vi "Read Element of Array.vi"(8 "error in (no error)":errorcluster, 10 "index":i32, 11 "parcour_Liste in":refnum<class "parcour_Liste.lvclass">) -> (0 "error out":errorcluster, 2 "Parcour_element.lvclass":refnum<class "Parcour_element.lvclass">, 3 "parcour_Liste out":refnum<class "parcour_Liste.lvclass">)   [LabVIEW 2019, in "parcour_Liste.lvclass"]
uses:
  parcour_Liste.lvclass
  parcour/Parcour_element.lvclass
  parcour_Liste.lvclass/parcour_Liste.ctl
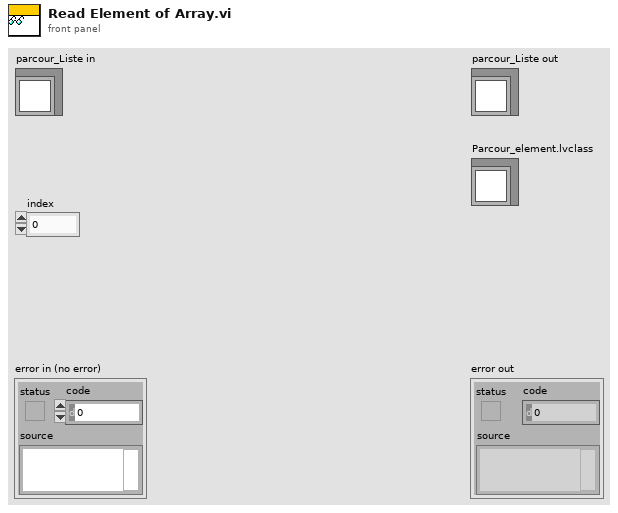
[diagram p1: front panel]
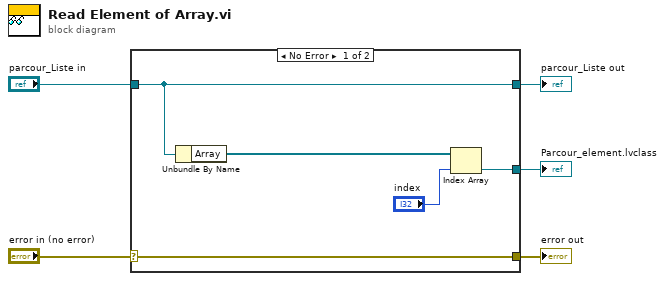
[diagram p0: block diagram]
diagram:
  n1 = case shown="No Error" "error in (no error)" {
    selector: "error in (no error)" -> [w10 w11]
    tunnel: [w10 w11] -> w4
    tunnel: [w9 w12] -> w2
    tunnel: "parcour_Liste in" -> [w9 w12]
    tunnel: [w6 _] -> w1
    frame No Error {
      n2 = Unbundle By Name(w9) -> ("Array"=w8:refnum<class "Parcour_element.lvclass">[])
      n3 = Index Array(array=w8, index="index") -> (element=w6:refnum<class "Parcour_element.lvclass">)
    }
    frame Error {
    }
  }
  "error out" <- w4
  "parcour_Liste out" <- w2
  "Parcour_element.lvclass" <- w1
